vi "SaveInFile.vi"(0 "path":path, 7 "pressureData":string[](array[string]), 9 "tempData":string, 11 "4071data":string[](array[string])) -> (4 "refnum out":refnum<file>, 6 "refnum out 2":refnum<file>, 8 "refnum out 3":refnum<file>, 15 "error out":errorcluster)   [LabVIEW 2019]
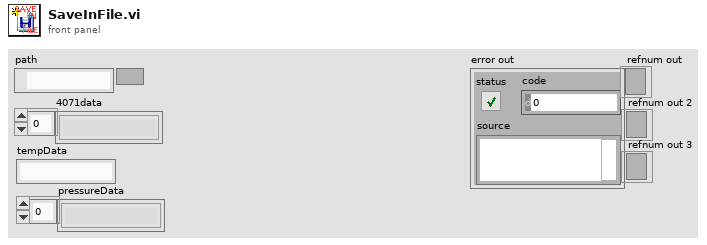
[diagram p1: front panel]
types:
  T1 = enum16{"open", "replace", "create", "open or create", "replace or create", "replace or create with confirmation"}
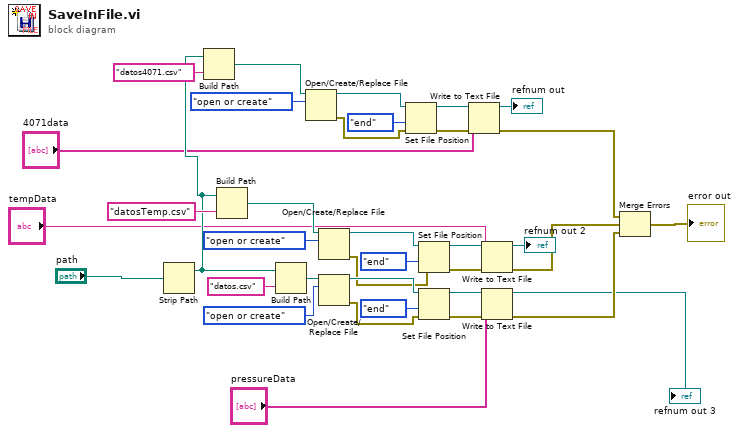
[diagram p0: block diagram]
diagram:
  n1 = Strip Path(path="path") -> (stripped path=w17:path)  [unwired: 1 out]
  n2 = Build Path(base path=w17, name or relative path="datos4071.csv") -> (appended path=w21:path)
  n3 = Build Path(base path=w17, name or relative path="datosTemp.csv") -> (appended path=w35:path)
  n4 = Build Path(base path=w17, name or relative path="datos.csv") -> (appended path=w32:path)
  n5 = Open/Create/Replace File(file path (use dialog)=w21, operation (0:open)=T1."open or create") -> (refnum out=w20:refnum<file>, error out=w14:errorcluster)  [unwired: 4 in, 1 out]
  n6 = Open/Create/Replace File(file path (use dialog)=w35, operation (0:open)=T1."open or create") -> (refnum out=w34:refnum<file>, error out=w13:errorcluster)  [unwired: 4 in, 1 out]
  n7 = Open/Create/Replace File(file path (use dialog)=w32, operation (0:open)=T1."open or create") -> (refnum out=w29:refnum<file>, error out=w12:errorcluster)  [unwired: 4 in, 1 out]
  n8 = Set File Position(refnum=w20, from (0:start)=enum16{"start", "end", "current"}."end", error in=w14) -> (refnum out=w22:refnum<file>, error out=w15:errorcluster)  [unwired: 1 in]
  n9 = Set File Position(refnum=w34, from (0:start)=enum16{"start", "end", "current"}."end", error in=w13) -> (refnum out=w36:refnum<file>, error out=w33:errorcluster)  [unwired: 1 in]
  n10 = Set File Position(refnum=w29, from (0:start)=enum16{"start", "end", "current"}."end", error in=w12) -> (refnum out=w30:refnum<file>, error out=w31:errorcluster)  [unwired: 1 in]
  n11 = Write to Text File(file (use dialog)=w22, text="4071data", error in=w15) -> (refnum out=→"refnum out":refnum<file>, error out=w5:errorcluster)  [unwired: 1 in, 1 out]
  n12 = Write to Text File(file (use dialog)=w36, text="tempData", error in=w33) -> (refnum out=→"refnum out 2":refnum<file>, error out=w6:errorcluster)  [unwired: 1 in, 1 out]
  n13 = Write to Text File(file (use dialog)=w30, text="pressureData", error in=w31) -> (refnum out=→"refnum out 3":refnum<file>, error out=w7:errorcluster)  [unwired: 1 in, 1 out]
  n14 = Merge Errors(w5, w6, w7) -> (→"error out":errorcluster)
